vi "解一元二次方程.vi"   [LabVIEW 2018]
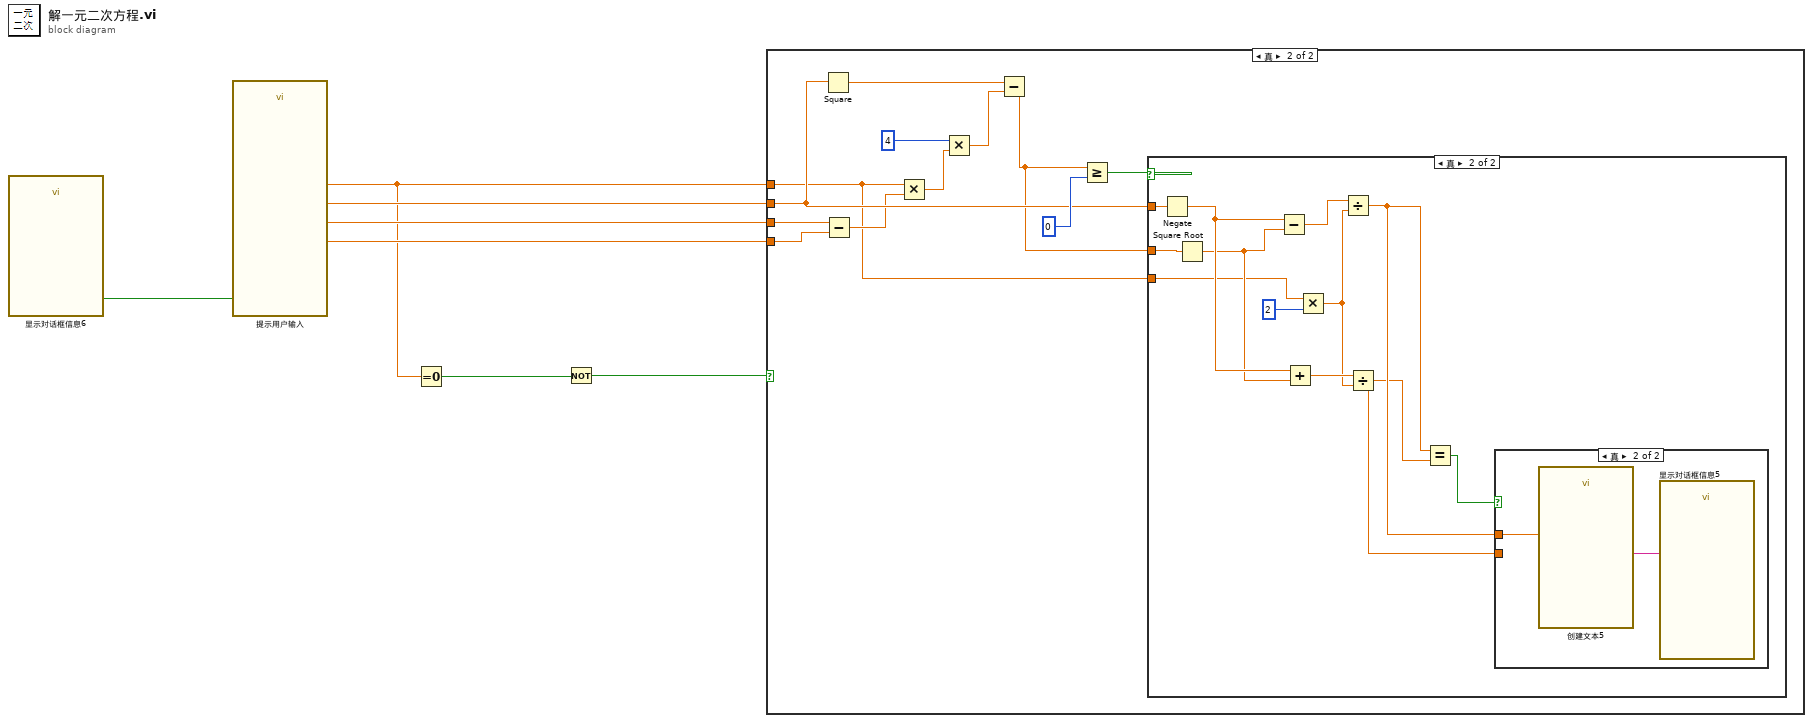
[diagram p0: block diagram]
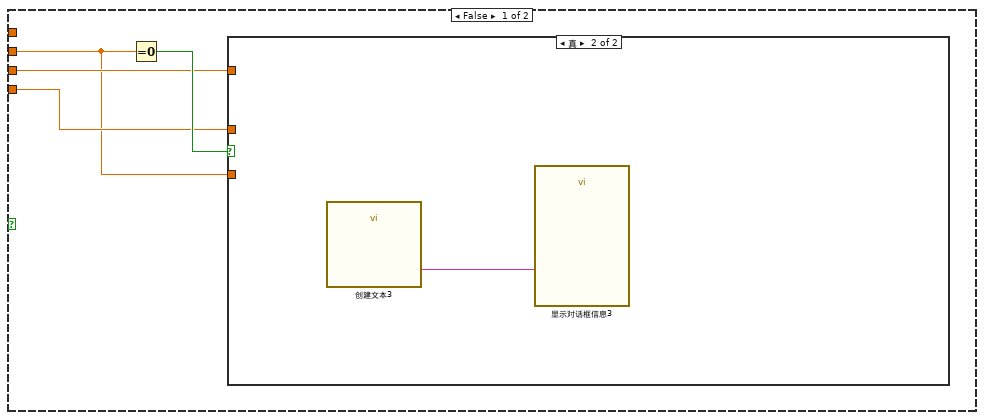
[diagram p2: hidden frame]
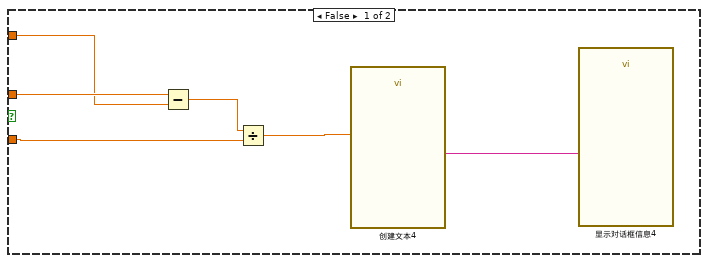
[diagram p3: hidden frame]
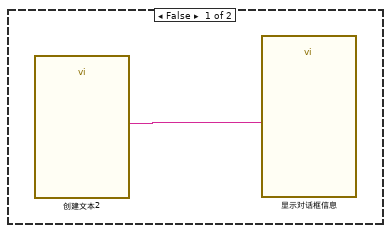
[diagram p4: hidden frame]
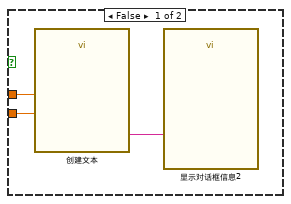
[diagram p5: hidden frame]
diagram:
  n1 = call "显示对话框信息6"() -> ("确定"=w1:bool)  [unwired: 10 in, 1 out]
  n2 = call "提示用户输入"("Enable"=w1) -> ("D"=w5:dbl, "C"=w6:dbl, "B"=w7:dbl, "A"=w4:dbl)  [unwired: 13 in, 2 out]
  n3 = Equal To 0?(x=w4) -> (x = 0?=w3:bool)
  n4 = Not(x=w3) -> (.not. x?=w2:bool)
  n5 = case shown="真" w2 {
    tunnel: w7 -> [w8 w25]
    tunnel: w6 -> [w9 w22]
    tunnel: w5 -> [w10 w21]
    tunnel: w4 -> [_ w19]
    frame False {
      n6 = Equal To 0?(x=w8) -> (x = 0?=w11:bool)
      n7 = case shown="真" w11 {
        tunnel: w10 -> [w17 _]
        tunnel: w9 -> [w16 _]
        tunnel: w8 -> [w14 _]
        frame False {
          n8 = Subtract(x=w17, y=w16) -> (x-y=w15:dbl)
          n9 = Divide(x=w15, y=w14) -> (x/y=w13:dbl)
          n10 = call "创建文本4"("a"=w13) -> ("Result"=w12:string)  [unwired: 13 in, 1 out]
          n11 = call "显示对话框信息4"("Message"=w12) -> ()  [unwired: 9 in, 2 out]
        }
        frame True {
          n12 = call "创建文本3"() -> ("Result"=w18:string)  [unwired: 14 in, 1 out]
          n13 = call "显示对话框信息3"("Message"=w18) -> ()  [unwired: 9 in, 2 out]
        }
      }
    }
    frame True {
      n14 = Square(x=w25) -> (x^2=w29:dbl)
      n15 = Subtract(x=w22, y=w21) -> (x-y=w20:dbl)
      n16 = Multiply(x=w19, y=w20) -> (x*y=w23:dbl)
      n17 = Multiply(x=4, y=w23) -> (x*y=w28:dbl)
      n18 = Subtract(x=w29, y=w28) -> (x-y=w24:dbl)
      n19 = Greater Or Equal?(x=w24, y=0) -> (x >= y?=w26:bool)
      n20 = case shown="真" w26 {
        tunnel: w25 -> [_ w43]
        tunnel: w24 -> [_ w42]
        tunnel: w19 -> [_ w39]
        frame False {
          n21 = call "创建文本2"() -> ("Result"=w31:string)  [unwired: 14 in, 1 out]
          n22 = call "显示对话框信息"("Message"=w31) -> ()  [unwired: 9 in, 2 out]
        }
        frame True {
          n23 = Negate(x=w43) -> (-x=w41:dbl)
          n24 = Square Root(x=w42) -> (sqrt(x)=w40:dbl)
          n25 = Subtract(x=w41, y=w40) -> (x-y=w37:dbl)
          n26 = Add(x=w41, y=w40) -> (x+y=w36:dbl)
          n27 = Multiply(x=w39, y=2) -> (x*y=w35:dbl)
          n28 = Divide(x=w37, y=w35) -> (x/y=w33:dbl)
          n29 = Divide(x=w36, y=w35) -> (x/y=w32:dbl)
          n30 = Equal?(x=w33, y=w32) -> (x = y?=w34:bool)
          n31 = case shown="真" w34 {
            tunnel: w33 -> [w46 w47]
            tunnel: w32 -> [w45 _]
            frame False {
              n32 = call "创建文本"("A"=w46, "B"=w45) -> ("Result"=w44:string)  [unwired: 12 in, 1 out]
              n33 = call "显示对话框信息2"("Message"=w44) -> ()  [unwired: 9 in, 2 out]
            }
            frame True {
              n34 = call "创建文本5"("a"=w47) -> ("Result"=w48:string)  [unwired: 13 in, 1 out]
              n35 = call "显示对话框信息5"("Message"=w48) -> ()  [unwired: 9 in, 2 out]
            }
          }
        }
      }
    }
  }
